vi "Instantiate LV RT.vi"   [LabVIEW 2019, in "LV RT.lvclass"]
uses:
  LV RT.lvclass
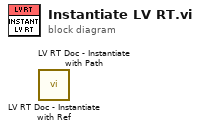
[diagram p0: block diagram]
diagram:
  n1 = call "LV RT Doc - Instantiate with Ref.vi"() -> ()  [unwired: 14 in, 2 out]
  n2 = call "LV RT Doc - Instantiate with Path.vi"() -> ()  [unwired: 14 in, 2 out]
